vi "SET_DEC.vi"(0 "TCP Network Connection in":refnum<k5>, 2 "N":u32=100, 5 "error in (no error)":errorcluster) -> (14 "TCP Network Connection out":refnum<k5>, 15 "DEC_STATUS":u8[](array[numeric]), 19 "error out":errorcluster)   [LabVIEW 2019]
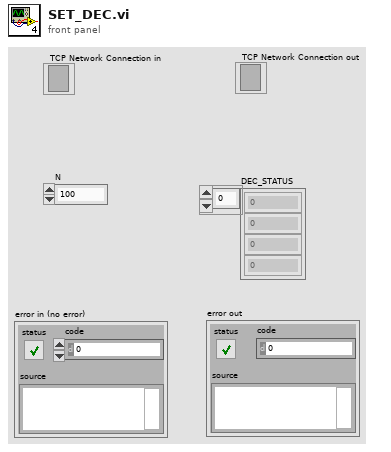
[diagram p1: front panel]
types:
  T1 = enum16{"big-endian, network order", "native, host order", "little-endian"}
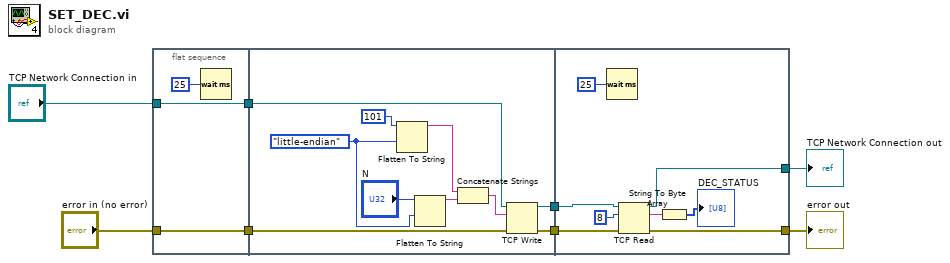
[diagram p0: block diagram]
diagram:
  n1 = flat-sequence {
    tunnel: [w10] -> w4
    tunnel: [w11] -> w3
    tunnel: "error in (no error)" -> [w11]
    tunnel: "TCP Network Connection in" -> [w10]
    tunnel: w4 -> [w21]
    tunnel: w3 -> [w20]
    tunnel: [w19] -> w2
    tunnel: [w18] -> w1
    tunnel: [w26] -> w6
    tunnel: [w27] -> w5
    tunnel: w2 -> [w29]
    tunnel: w1 -> [w28]
    frame #0 {
      n2 = Wait (ms)(milliseconds to wait=u32 25) -> ()  [unwired: 1 out]
    }
    frame #1 {
      w16 = T1."little-endian" ("byte order (0:big-endian, network order)")
      n3 = Flatten To String(anything=u32 101 ("element"), byte order (0:big-endian, network order)=w16) -> (data string=w14:string)  [unwired: 2 in, 2 out]
      n4 = Flatten To String(anything="N", byte order (0:big-endian, network order)=w16) -> (data string=w17:string)  [unwired: 2 in, 2 out]
      n5 = Concatenate Strings(w14, w17) -> (w13:string)
      n6 = TCP Write(connection ID=w21, data in=w13, error in (no error)=w20) -> (connection ID out=w19:refnum<k5>, error out=w18:errorcluster)  [unwired: 1 in, 1 out]
    }
    frame #2 {
      n7 = Wait (ms)(milliseconds to wait=u32 25) -> ()  [unwired: 1 out]
      n8 = TCP Read(connection ID=w29, bytes to read=8, error in (no error)=w28) -> (connection ID out=w27:refnum<k5>, data out=w23:string, error out=w26:errorcluster)  [unwired: 2 in]
      n9 = String To Byte Array(string=w23) -> (unsigned byte array=→"DEC_STATUS":u8[])
    }
  }
  "error out" <- w6
  "TCP Network Connection out" <- w5
